vi "MoveMotor.vi"(8 "Proportional Gain":dbl, 11 "Teeth":dbl) -> ()   [LabVIEW 2017]
panel:
  in  "stop":bool
  out "Error":dbl
  out "Tooth Count (Doubled)":dbl
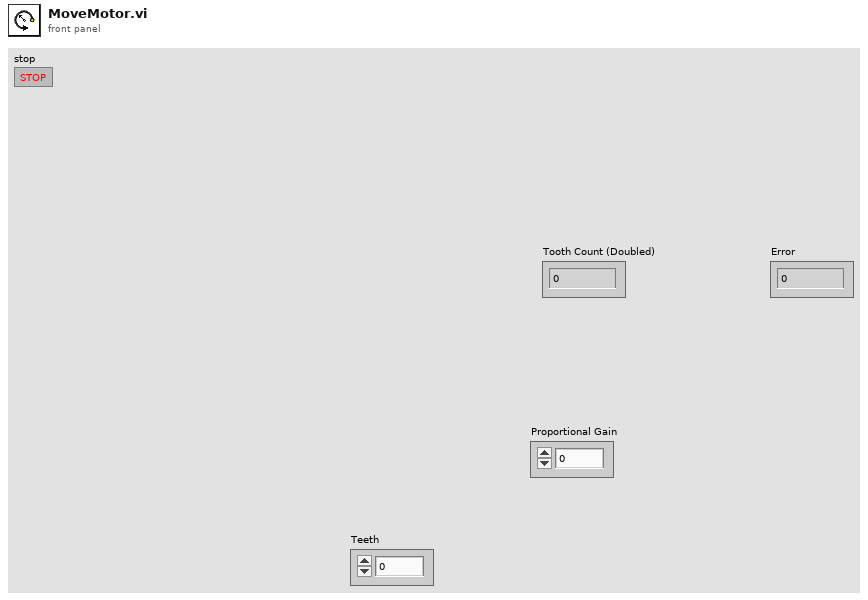
[diagram p1: front panel]
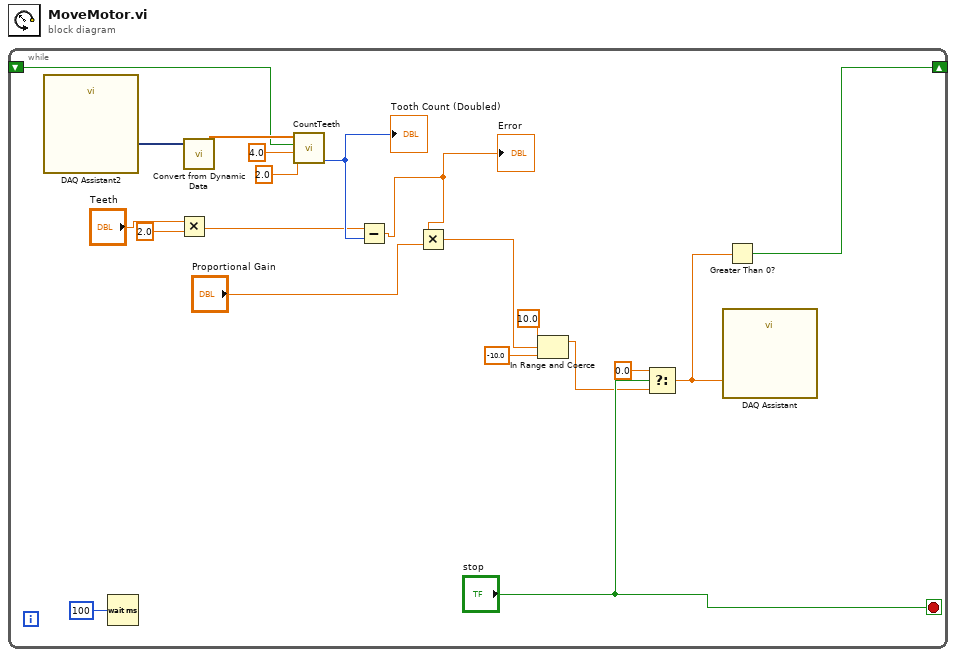
[diagram p0: block diagram]
diagram:
  n1 = while {
    shift-right: [w2] -> _
    shift-left: _ -> [w1]
    stop <- "stop" stop-if-true
    n2 = call "DAQ Assistant2"() -> ("data"=w20:dynamicdata)  [unwired: 17 in, 2 out]
    n3 = Wait (ms)(milliseconds to wait=u32 100) -> ()  [unwired: 1 out]
    n4 = Multiply(x="Teeth", y=2.0) -> (x*y=w13:dbl)
    n5 = call "Convert from Dynamic Data"("Dynamic Data Type"=w20) -> ("Array"=w19:dbl[])  [unwired: 3 in]
    n6 = call "CountTeeth.vi"("Falling Threshold"=2.0, "Rising Threshold"=4.0, "Direction"=w1, "Array"=w19) -> ("Gear Count"=w16:i32)  [unwired: 7 in]
    "Tooth Count (Doubled)" <- w16
    n7 = Subtract(x=w13, y=w16) -> (x-y=w11:dbl)
    "Error" <- w11
    n8 = Multiply(x=w11, y="Proportional Gain") -> (x*y=w10:dbl)
    n9 = In Range and Coerce(upper limit=10.0, x=w10, lower limit=-10.0) -> (coerced(x)=w5:dbl)  [unwired: 1 out]
    n10 = Select(t=0.0, s="stop", f=w5) -> (s? t:f=w3:dbl)
    n11 = call "DAQ Assistant"("data"=w3) -> ()  [unwired: 17 in, 2 out]
    n12 = Greater Than 0?(x=w3) -> (x > 0?=w2:bool)
  }
